vi "Execute Process Step.vi"(8 "error in (no error)":errorcluster, 11 "Process Model in":refnum<class "Process Model.lvclass">) -> (0 "error out":errorcluster, 3 "Process Model out":refnum<class "Process Model.lvclass">)   [LabVIEW 2017, in "Car Wash.lvlib" / "Process Model.lvlib" / "Process Model.lvclass"]
uses:
  Process Model.lvclass
  <vilib>/gpm_packages/@cs/test-executive/Source/Test Executive/TestExecutive Ref/TestExecutive Ref.lvclass
  <vilib>/ActorFramework/Actor/Actor.lvclass
  <vilib>/gpm_packages/@cs/test-executive/Source/Test Executive/Executioner/Executioner.lvclass
  iProcess Step Model/iProcess Step Model/iProcess Step Model.lvclass
  <vilib>/gpm_packages/@cs/mva-core/Source/IModel/IModel/IModel.lvclass
  C:/Program Files/National Instruments/LabVIEW 2017/vi.lib/gpm_packages/@cs/mva-core/Source/IObserver/IObserver/IObserver.lvclass
  C:/Program Files/National Instruments/LabVIEW 2017/vi.lib/ActorFramework/Actor/Actor.lvclass
  D:/Project/General VIs/Process/iProcess Model/iProcess Model/iProcess Model.lvclass
  C:/Program Files/National Instruments/LabVIEW 2017/vi.lib/gpm_packages/@cs/mva-core/Source/IModel/IModel/IModel.lvclass
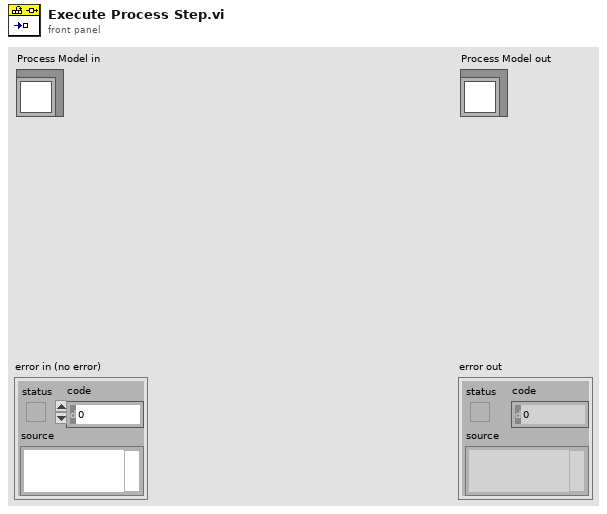
[diagram p1: front panel]
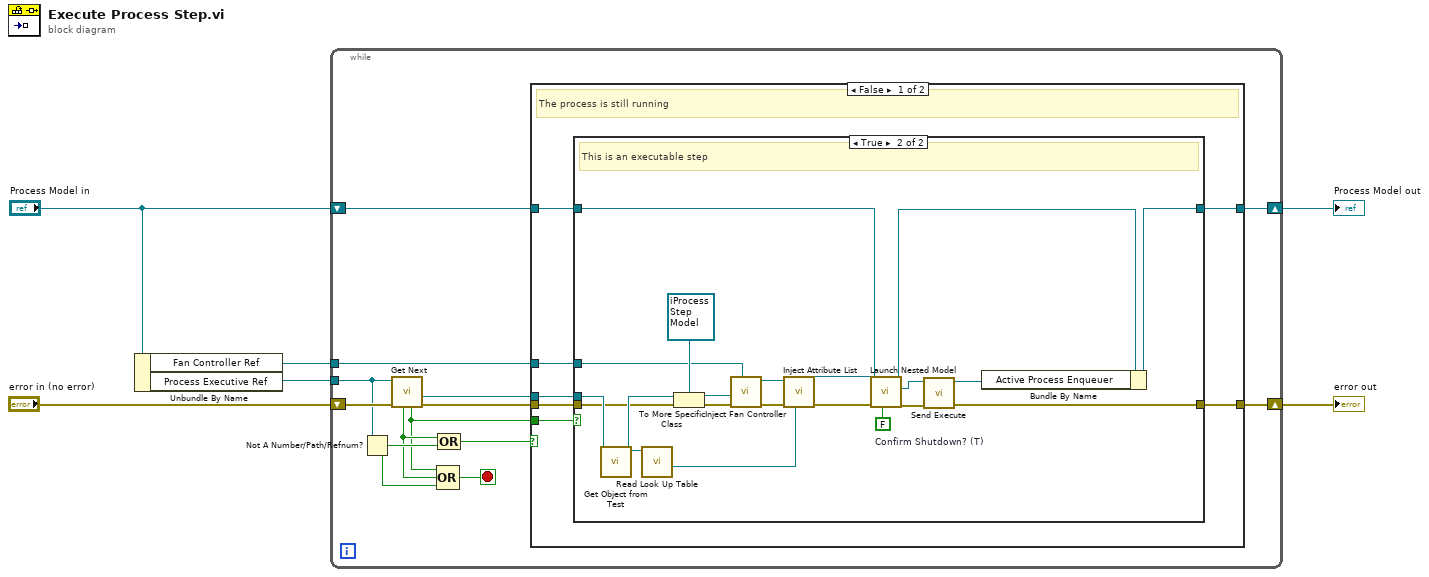
[diagram p0: block diagram]
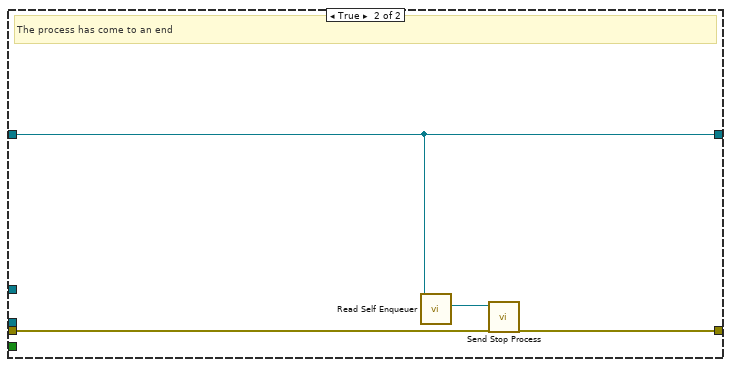
[diagram p3: hidden frame]
diagram:
  n1 = Unbundle By Name("Process Model in") -> ("Fan Controller Ref"=w1:refnum<data-value>, "Process Executive Ref"=w2:refnum<data-value>)
  n2 = while {
    shift-right: [w15] -> w6
    shift-left: "Process Model in" -> [w16]
    shift-right: [w13] -> w4
    shift-left: "error in (no error)" -> [w19]
    tunnel: w2 -> [w18]
    tunnel: w1 -> [w7]
    stop <- w17 stop-if-true
    n3 = Not A Number/Path/Refnum?(number/path/refnum=w18) -> (NaN/Path/Refnum?=w12:bool)
    n4 = call <vilib>:"Get Next.vi"("error in (no error)"=w19, "Test Executive Ref"=w18) -> ("error out"=w14:errorcluster, "Test"=w9:refnum<class "Executioner.lvclass">, "Found"=w8:bool, "Complete"=w11:bool)  [unwired: 3 in, 3 out]
    n5 = Compound Arithmetic op=OR(w8, w11, w12) -> (w17:bool)
    n6 = Compound Arithmetic op=OR(w11, w12) -> (w10:bool)
    n7 = case shown="False" w10 {
      tunnel: [w24 w53] -> w15
      tunnel: w16 -> [w25 w53]
      tunnel: [w22 w50] -> w13
      tunnel: w14 -> [w23 w51]
      tunnel: w9 -> [w21 _]
      tunnel: w8 -> [w26 _]
      tunnel: w7 -> [w20 _]
      frame False {
        # "The process is still running"
        n8 = case shown="True" w26 {
          tunnel: [w28 w39] -> w24
          tunnel: w25 -> [w28 w43]
          tunnel: [w27 w35] -> w22
          tunnel: w23 -> [w27 w46]
          tunnel: w21 -> [_ w49]
          tunnel: w20 -> [_ w30]
          frame False {
            # "This is a flow control process"
          }
          frame True {
            w29 = FALSE  # Confirm Shutdown? (T)
            # "This is an executable step"
            n9 = call <vilib>:"Get Object from Test.vi"("Executioner in"=w49) -> ("Test"=w47:refnum<class>, "Executioner out"=w48:refnum<class "Executioner.lvclass">)  [unwired: 9 in]
            n10 = call <vilib>:"Read Look Up Table.vi"("Executioner in"=w48) -> ("Attributes Ref"=w44:refnum<data-value>)  [unwired: 9 in, 1 out]
            n11 = To More Specific Class(target class=refnum<class "iProcess Step Model.lvclass"> refnum ("iProcess Step Model.lvclass"), reference=w47, error in=w46) -> (specific class reference=w32:refnum<class "iProcess Step Model.lvclass">, error out=w34:errorcluster)
            n12 = call-dynamic "Inject Fan Controller.vi"("Fan Controller Ref"=w30, "error in (no error)"=w34, "iProcess Step Model in"=w32) -> ("error out"=w33:errorcluster, "iProcess Step Model out"=w31:refnum<class "iProcess Step Model.lvclass">)  [unwired: 7 in]
            n13 = call-dynamic "Inject Attribute List.vi"("Attributes Ref"=w44, "error in (no error)"=w33, "iProcess Step Model in"=w31) -> ("error out"=w42:errorcluster, "iProcess Step Model out"=w41:refnum<class "iProcess Step Model.lvclass">)  [unwired: 7 in]
            n14 = call-dynamic "Launch Nested Model.vi"("Confirm Shutdown? (T)"=w29, "error in (no error)"=w42, "Model to Launch"=w41, "IModel in"=w43) -> ("error out"=w36:errorcluster, "Nested Model Enqueuer"=w38:refnum<class "Message Enqueuer.lvclass">, "IModel out"=w40:refnum<class "Process Model.lvclass">)  [unwired: 5 in]
            n15 = call "Send Execute.vi"("error in (no error)"=w36, "Message Enqueuer"=w38) -> ("error out"=w35:errorcluster, "Message Enqueuer out"=w37:refnum<class "Message Enqueuer.lvclass">)  [unwired: 8 in]
            n16 = Bundle By Name(cluster=w40, "Active Process Enqueuer"=w37) -> (w39:refnum<class "Process Model.lvclass">)
          }
        }
      }
      frame True {
        # "The process has come to an end"
        n17 = call <vilib>:"Read Self Enqueuer.vi"("Actor"=w53) -> ("Self Enqueuer"=w52:refnum<class "Message Enqueuer.lvclass">)  [unwired: 10 in]
        n18 = call "Send Stop Process.vi"("error in (no error)"=w51, "Message Enqueuer"=w52) -> ("error out"=w50:errorcluster)  [unwired: 8 in, 1 out]
      }
    }
  }
  "error out" <- w4
  "Process Model out" <- w6
